vi "Lab Panel V5.25.1.vi"() -> ()   [LabVIEW 2013] (continued)
                    n1123 = Unbundle(w2133) -> ("CYCLE"=w2138:dbl)  [unwired: 2 out]
                    n1124 = Increment(x=w2130) -> (x+1=w2131:dbl)
                    n1125 = Greater Or Equal?(x=w2138, y=w2131) -> (x >= y?=w2140:bool)
                    n1126 = case shown="True" w2140 {
                      tunnel: w2135 -> [w2150 _]
                      tunnel: w2134 -> [w2149 _]
                      tunnel: w2133 -> [w2148 _]
                      tunnel: w2132 -> [w2147 _]
                      frame True {
                        n1127 = stacked-sequence {
                          tunnel: w2150 -> [w2154 _]
                          tunnel: w2149 -> [w2152 w2158]
                          tunnel: w2148 -> [_ w2161]
                          tunnel: w2147 -> [w2151 _]
                          frame #0 {
                            n1128 = Build Array(w2152) -> (w2155:string[])
                            n1129 = Build Array(w2154) -> (w2153:dbl[])
                            n1130 = TDMS Write(0:w2151, 5:"TEST PASS", 7:w2155, 9:w2153) -> (15:w2157:errorcluster)  [unwired: 2 in, 3 out]
                            n1131 = local write "data file error"(w2157) -> ()
                          }
                          frame #1 {
                            n1132 = Bundle(cluster=w2161, "STATUS"=w2158) -> (w2159:T4)  [unwired: 2 in]
                            n1133 = local write "RESULT LAB01-1"(TRUE) -> ()
                            n1134 = local write "DISP LAB01-1"(w2159) -> ()
                          }
                        }
                      }
                      frame False {
                      }
                    }
                  }
                }
              }
              frame #1 {
                # "LAB01-2"
                n1135 = Less?(x=w2162, y=2) -> (x < y?=w2165:bool)
                n1136 = local read "DISP LAB01-2"() -> (w2167:T4)
                n1137 = Unbundle(w2167) -> ("STATUS"=w2168:string)  [unwired: 2 out]
                n1138 = Equal?(x=w2168, y="RUN") -> (x = y?=w2164:bool)
                n1139 = And(x=w2164, y=w2165) -> (x .and. y?=w2163:bool)
                n1140 = case shown="True" w2163 {
                  tunnel: w2167 -> [_ w2173]
                  tunnel: w2162 -> [_ w2177]
                  frame False {
                  }
                  frame True {
                    n1141 = local read "SET LAB01-2"() -> (w2179:T5)
                    n1142 = local read "TDMS LAB01-2"() -> (w2172:refnum<k34>)
                    n1143 = Unbundle(w2179) -> ("CYCLES"=w2170:dbl, "T-RISE mins"=w2176:dbl)  [unwired: 3 out]
                    n1144 = case shown="\"T-RISE TEST\"" w2177 {
                      tunnel: w2176 -> [_ _ w2186]
                      tunnel: [w2181 w2183 w2186] -> w2175
                      tunnel: w2170 -> [w2181 w2183 _]
                      tunnel: ["CHART PASS" "CYCLE PASS" "T-RISE PASS"] -> w2174
                      frame "CHART TEST", Default {
                      }
                      frame "CYCLE TEST" {
                      }
                      frame "T-RISE TEST" {
                      }
                    }
                    n1145 = Unbundle(w2173) -> ("CYCLE"=w2178:dbl)  [unwired: 2 out]
                    n1146 = Increment(x=w2170) -> (x+1=w2171:dbl)
                    n1147 = Greater Or Equal?(x=w2178, y=w2171) -> (x >= y?=w2180:bool)
                    n1148 = case shown="True" w2180 {
                      tunnel: w2175 -> [w2190 _]
                      tunnel: w2174 -> [w2189 _]
                      tunnel: w2173 -> [w2188 _]
                      tunnel: w2172 -> [w2187 _]
                      frame True {
                        n1149 = stacked-sequence {
                          tunnel: w2190 -> [w2194 _]
                          tunnel: w2189 -> [w2192 w2198]
                          tunnel: w2188 -> [_ w2201]
                          tunnel: w2187 -> [w2191 _]
                          frame #0 {
                            n1150 = Build Array(w2192) -> (w2195:string[])
                            n1151 = Build Array(w2194) -> (w2193:dbl[])
                            n1152 = TDMS Write(0:w2191, 5:"TEST PASS", 7:w2195, 9:w2193) -> (15:w2197:errorcluster)  [unwired: 2 in, 3 out]
                            n1153 = local write "data file error"(w2197) -> ()
                          }
                          frame #1 {
                            n1154 = Bundle(cluster=w2201, "STATUS"=w2198) -> (w2199:T4)  [unwired: 2 in]
                            n1155 = local write "RESULT LAB01-2"(TRUE) -> ()
                            n1156 = local write "DISP LAB01-2"(w2199) -> ()
                          }
                        }
                      }
                      frame False {
                      }
                    }
                  }
                }
              }
              frame #2 {
                # "LAB02-1"
                n1157 = Less?(x=w2202, y=2) -> (x < y?=w2205:bool)
                n1158 = local read "DISP LAB02-1"() -> (w2207:T4)
                n1159 = Unbundle(w2207) -> ("STATUS"=w2208:string)  [unwired: 2 out]
                n1160 = Equal?(x=w2208, y="RUN") -> (x = y?=w2204:bool)
                n1161 = And(x=w2204, y=w2205) -> (x .and. y?=w2203:bool)
                n1162 = case shown="True" w2203 {
                  tunnel: w2207 -> [_ w2213]
                  tunnel: w2202 -> [_ w2217]
                  frame False {
                  }
                  frame True {
                    n1163 = local read "SET LAB02-1"() -> (w2219:T5)
                    n1164 = local read "TDMS LAB02-1"() -> (w2212:refnum<k34>)
                    n1165 = Unbundle(w2213) -> ("CYCLE"=w2218:dbl)  [unwired: 2 out]
                    n1166 = Unbundle(w2219) -> ("CYCLES"=w2210:dbl, "T-RISE mins"=w2216:dbl)  [unwired: 3 out]
                    n1167 = case shown="\"T-RISE TEST\"" w2217 {
                      tunnel: w2216 -> [_ _ w2226]
                      tunnel: [w2221 w2223 w2226] -> w2215
                      tunnel: w2210 -> [w2221 w2223 _]
                      tunnel: ["CHART PASS" "CYCLE PASS" "T-RISE PASS"] -> w2214
                      frame "CHART TEST", Default {
                      }
                      frame "CYCLE TEST" {
                      }
                      frame "T-RISE TEST" {
                      }
                    }
                    n1168 = Increment(x=w2210) -> (x+1=w2211:dbl)
                    n1169 = Greater Or Equal?(x=w2218, y=w2211) -> (x >= y?=w2220:bool)
                    n1170 = case shown="True" w2220 {
                      tunnel: w2215 -> [w2230 _]
                      tunnel: w2214 -> [w2229 _]
                      tunnel: w2213 -> [w2228 _]
                      tunnel: w2212 -> [w2227 _]
                      frame True {
                        n1171 = stacked-sequence {
                          tunnel: w2230 -> [w2234 _]
                          tunnel: w2229 -> [w2232 w2238]
                          tunnel: w2228 -> [_ w2241]
                          tunnel: w2227 -> [w2231 _]
                          frame #0 {
                            n1172 = Build Array(w2232) -> (w2235:string[])
                            n1173 = Build Array(w2234) -> (w2233:dbl[])
                            n1174 = TDMS Write(0:w2231, 5:"TEST PASS", 7:w2235, 9:w2233) -> (15:w2237:errorcluster)  [unwired: 2 in, 3 out]
                            n1175 = local write "data file error"(w2237) -> ()
                          }
                          frame #1 {
                            n1176 = Bundle(cluster=w2241, "STATUS"=w2238) -> (w2239:T4)  [unwired: 2 in]
                            n1177 = local write "RESULT LAB02-1"(TRUE) -> ()
                            n1178 = local write "DISP LAB02-1"(w2239) -> ()
                          }
                        }
                      }
                      frame False {
                      }
                    }
                  }
                }
              }
              frame #3 {
                # "LAB02-2"
                n1179 = Less?(x=w2242, y=2) -> (x < y?=w2245:bool)
                n1180 = local read "DISP LAB02-2"() -> (w2247:T4)
                n1181 = Unbundle(w2247) -> ("STATUS"=w2248:string)  [unwired: 2 out]
                n1182 = Equal?(x=w2248, y="RUN") -> (x = y?=w2244:bool)
                n1183 = And(x=w2244, y=w2245) -> (x .and. y?=w2243:bool)
                n1184 = case shown="True" w2243 {
                  tunnel: w2247 -> [_ w2253]
                  tunnel: w2242 -> [_ w2257]
                  frame False {
                  }
                  frame True {
                    n1185 = local read "SET LAB02-2"() -> (w2259:T5)
                    n1186 = local read "TDMS LAB02-2"() -> (w2252:refnum<k34>)
                    n1187 = Unbundle(w2253) -> ("CYCLE"=w2258:dbl)  [unwired: 2 out]
                    n1188 = Unbundle(w2259) -> ("CYCLES"=w2250:dbl, "T-RISE mins"=w2256:dbl)  [unwired: 3 out]
                    n1189 = case shown="\"T-RISE TEST\"" w2257 {
                      tunnel: w2256 -> [_ _ w2266]
                      tunnel: [w2261 w2263 w2266] -> w2255
                      tunnel: w2250 -> [w2261 w2263 _]
                      tunnel: ["CHART PASS" "CYCLE PASS" "T-RISE PASS"] -> w2254
                      frame "CHART TEST", Default {
                      }
                      frame "CYCLE TEST" {
                      }
                      frame "T-RISE TEST" {
                      }
                    }
                    n1190 = Increment(x=w2250) -> (x+1=w2251:dbl)
                    n1191 = Greater Or Equal?(x=w2258, y=w2251) -> (x >= y?=w2260:bool)
                    n1192 = case shown="True" w2260 {
                      tunnel: w2255 -> [w2270 _]
                      tunnel: w2254 -> [w2269 _]
                      tunnel: w2253 -> [w2268 _]
                      tunnel: w2252 -> [w2267 _]
                      frame True {
                        n1193 = stacked-sequence {
                          tunnel: w2270 -> [w2274 _]
                          tunnel: w2269 -> [w2272 w2278]
                          tunnel: w2268 -> [_ w2281]
                          tunnel: w2267 -> [w2271 _]
                          frame #0 {
                            n1194 = Build Array(w2272) -> (w2275:string[])
                            n1195 = Build Array(w2274) -> (w2273:dbl[])
                            n1196 = TDMS Write(0:w2271, 5:"TEST PASS", 7:w2275, 9:w2273) -> (15:w2277:errorcluster)  [unwired: 2 in, 3 out]
                            n1197 = local write "data file error"(w2277) -> ()
                          }
                          frame #1 {
                            n1198 = Bundle(cluster=w2281, "STATUS"=w2278) -> (w2279:T4)  [unwired: 2 in]
                            n1199 = local write "RESULT LAB02-2"(TRUE) -> ()
                            n1200 = local write "DISP LAB02-2"(w2279) -> ()
                          }
                        }
                      }
                      frame False {
                      }
                    }
                  }
                }
              }
              frame #4 {
                # "LAB03-1"
                n1201 = Less?(x=w2282, y=2) -> (x < y?=w2285:bool)
                n1202 = local read "DISP LAB03-1"() -> (w2287:T4)
                n1203 = Unbundle(w2287) -> ("STATUS"=w2288:string)  [unwired: 2 out]
                n1204 = Equal?(x=w2288, y="RUN") -> (x = y?=w2284:bool)
                n1205 = And(x=w2284, y=w2285) -> (x .and. y?=w2283:bool)
                n1206 = case shown="True" w2283 {
                  tunnel: w2287 -> [_ w2293]
                  tunnel: w2282 -> [_ w2297]
                  frame False {
                  }
                  frame True {
                    n1207 = local read "SET LAB03-1"() -> (w2299:T5)
                    n1208 = local read "TDMS LAB03-1"() -> (w2292:refnum<k34>)
                    n1209 = Unbundle(w2293) -> ("CYCLE"=w2298:dbl)  [unwired: 2 out]
                    n1210 = Unbundle(w2299) -> ("CYCLES"=w2290:dbl, "T-RISE mins"=w2296:dbl)  [unwired: 3 out]
                    n1211 = case shown="\"T-RISE TEST\"" w2297 {
                      tunnel: w2296 -> [_ _ w2306]
                      tunnel: [w2301 w2303 w2306] -> w2295
                      tunnel: w2290 -> [w2301 w2303 _]
                      tunnel: ["CHART PASS" "CYCLE PASS" "T-RISE PASS"] -> w2294
                      frame "CHART TEST", Default {
                      }
                      frame "CYCLE TEST" {
                      }
                      frame "T-RISE TEST" {
                      }
                    }
                    n1212 = Increment(x=w2290) -> (x+1=w2291:dbl)
                    n1213 = Greater Or Equal?(x=w2298, y=w2291) -> (x >= y?=w2300:bool)
                    n1214 = case shown="True" w2300 {
                      tunnel: w2295 -> [w2310 _]
                      tunnel: w2294 -> [w2309 _]
                      tunnel: w2293 -> [w2308 _]
                      tunnel: w2292 -> [w2307 _]
                      frame True {
                        n1215 = stacked-sequence {
                          tunnel: w2310 -> [w2314 _]
                          tunnel: w2309 -> [w2312 w2318]
                          tunnel: w2308 -> [_ w2321]
                          tunnel: w2307 -> [w2311 _]
                          frame #0 {
                            n1216 = Build Array(w2312) -> (w2315:string[])
                            n1217 = Build Array(w2314) -> (w2313:dbl[])
                            n1218 = TDMS Write(0:w2311, 5:"TEST PASS", 7:w2315, 9:w2313) -> (15:w2317:errorcluster)  [unwired: 2 in, 3 out]
                            n1219 = local write "data file error"(w2317) -> ()
                          }
                          frame #1 {
                            n1220 = Bundle(cluster=w2321, "STATUS"=w2318) -> (w2319:T4)  [unwired: 2 in]
                            n1221 = local write "RESULT LAB03-1"(TRUE) -> ()
                            n1222 = local write "DISP LAB03-1"(w2319) -> ()
                          }
                        }
                      }
                      frame False {
                      }
                    }
                  }
                }
              }
              frame #5 {
                # "LAB03-2"
                n1223 = Less?(x=w2322, y=2) -> (x < y?=w2325:bool)
                n1224 = local read "DISP LAB03-2"() -> (w2327:T4)
                n1225 = Unbundle(w2327) -> ("STATUS"=w2328:string)  [unwired: 2 out]
                n1226 = Equal?(x=w2328, y="RUN") -> (x = y?=w2324:bool)
                n1227 = And(x=w2324, y=w2325) -> (x .and. y?=w2323:bool)
                n1228 = case shown="True" w2323 {
                  tunnel: w2327 -> [_ w2333]
                  tunnel: w2322 -> [_ w2337]
                  frame False {
                  }
                  frame True {
                    n1229 = local read "SET LAB03-2"() -> (w2339:T5)
                    n1230 = local read "TDMS LAB03-2"() -> (w2332:refnum<k34>)
                    n1231 = Unbundle(w2333) -> ("CYCLE"=w2338:dbl)  [unwired: 2 out]
                    n1232 = Unbundle(w2339) -> ("CYCLES"=w2330:dbl, "T-RISE mins"=w2336:dbl)  [unwired: 3 out]
                    n1233 = case shown="\"T-RISE TEST\"" w2337 {
                      tunnel: w2336 -> [_ _ w2346]
                      tunnel: [w2341 w2343 w2346] -> w2335
                      tunnel: w2330 -> [w2341 w2343 _]
                      tunnel: ["CHART PASS" "CYCLE PASS" "T-RISE PASS"] -> w2334
                      frame "CHART TEST", Default {
                      }
                      frame "CYCLE TEST" {
                      }
                      frame "T-RISE TEST" {
                      }
                    }
                    n1234 = Increment(x=w2330) -> (x+1=w2331:dbl)
                    n1235 = Greater Or Equal?(x=w2338, y=w2331) -> (x >= y?=w2340:bool)
                    n1236 = case shown="True" w2340 {
                      tunnel: w2335 -> [w2350 _]
                      tunnel: w2334 -> [w2349 _]
                      tunnel: w2333 -> [w2348 _]
                      tunnel: w2332 -> [w2347 _]
                      frame True {
                        n1237 = stacked-sequence {
                          tunnel: w2350 -> [w2354 _]
                          tunnel: w2349 -> [w2352 w2358]
                          tunnel: w2348 -> [_ w2361]
                          tunnel: w2347 -> [w2351 _]
                          frame #0 {
                            n1238 = Build Array(w2352) -> (w2355:string[])
                            n1239 = Build Array(w2354) -> (w2353:dbl[])
                            n1240 = TDMS Write(0:w2351, 5:"TEST PASS", 7:w2355, 9:w2353) -> (15:w2357:errorcluster)  [unwired: 2 in, 3 out]
                            n1241 = local write "data file error"(w2357) -> ()
                          }
                          frame #1 {
                            n1242 = Bundle(cluster=w2361, "STATUS"=w2358) -> (w2359:T4)  [unwired: 2 in]
                            n1243 = local write "RESULT LAB03-2"(TRUE) -> ()
                            n1244 = local write "DISP LAB03-2"(w2359) -> ()
                          }
                        }
                      }
                      frame False {
                      }
                    }
                  }
                }
              }
              frame #6 {
                # "LAB04-1"
                n1245 = Less?(x=w2362, y=2) -> (x < y?=w2365:bool)
                n1246 = local read "DISP LAB04-1"() -> (w2367:T4)
                n1247 = Unbundle(w2367) -> ("STATUS"=w2368:string)  [unwired: 2 out]
                n1248 = Equal?(x=w2368, y="RUN") -> (x = y?=w2364:bool)
                n1249 = And(x=w2364, y=w2365) -> (x .and. y?=w2363:bool)
                n1250 = case shown="True" w2363 {
                  tunnel: w2367 -> [_ w2373]
                  tunnel: w2362 -> [_ w2377]
                  frame False {
                  }
                  frame True {
                    n1251 = local read "SET LAB04-1"() -> (w2379:T5)
                    n1252 = local read "TDMS LAB04-1"() -> (w2372:refnum<k34>)
                    n1253 = Unbundle(w2373) -> ("CYCLE"=w2378:dbl)  [unwired: 2 out]
                    n1254 = Unbundle(w2379) -> ("CYCLES"=w2370:dbl, "T-RISE mins"=w2376:dbl)  [unwired: 3 out]
                    n1255 = case shown="\"T-RISE TEST\"" w2377 {
                      tunnel: w2376 -> [_ _ w2386]
                      tunnel: [w2381 w2383 w2386] -> w2375
                      tunnel: w2370 -> [w2381 w2383 _]
                      tunnel: ["CHART PASS" "CYCLE PASS" "T-RISE PASS"] -> w2374
                      frame "CHART TEST", Default {
                      }
                      frame "CYCLE TEST" {
                      }
                      frame "T-RISE TEST" {
                      }
                    }
                    n1256 = Increment(x=w2370) -> (x+1=w2371:dbl)
                    n1257 = Greater Or Equal?(x=w2378, y=w2371) -> (x >= y?=w2380:bool)
                    n1258 = case shown="True" w2380 {
                      tunnel: w2375 -> [w2390 _]
                      tunnel: w2374 -> [w2389 _]
                      tunnel: w2373 -> [w2388 _]
                      tunnel: w2372 -> [w2387 _]
                      frame True {
                        n1259 = stacked-sequence {
                          tunnel: w2390 -> [w2394 _]
                          tunnel: w2389 -> [w2392 w2398]
                          tunnel: w2388 -> [_ w2401]
                          tunnel: w2387 -> [w2391 _]
                          frame #0 {
                            n1260 = Build Array(w2392) -> (w2395:string[])
                            n1261 = Build Array(w2394) -> (w2393:dbl[])
                            n1262 = TDMS Write(0:w2391, 5:"TEST PASS", 7:w2395, 9:w2393) -> (15:w2397:errorcluster)  [unwired: 2 in, 3 out]
                            n1263 = local write "data file error"(w2397) -> ()
                          }
                          frame #1 {
                            n1264 = Bundle(cluster=w2401, "STATUS"=w2398) -> (w2399:T4)  [unwired: 2 in]
                            n1265 = local write "RESULT LAB04-1"(TRUE) -> ()
                            n1266 = local write "DISP LAB04-1"(w2399) -> ()
                          }
                        }
                      }
                      frame False {
                      }
                    }
                  }
                }
              }
              frame #7 {
                # "LAB04-2"
                n1267 = Less?(x=w2402, y=2) -> (x < y?=w2405:bool)
                n1268 = local read "DISP LAB04-2"() -> (w2407:T4)
                n1269 = Unbundle(w2407) -> ("STATUS"=w2408:string)  [unwired: 2 out]
                n1270 = Equal?(x=w2408, y="RUN") -> (x = y?=w2404:bool)
                n1271 = And(x=w2404, y=w2405) -> (x .and. y?=w2403:bool)
                n1272 = case shown="True" w2403 {
                  tunnel: w2407 -> [_ w2413]
                  tunnel: w2402 -> [_ w2417]
                  frame False {
                  }
                  frame True {
                    n1273 = local read "SET LAB04-2"() -> (w2419:T5)
                    n1274 = local read "TDMS LAB04-2"() -> (w2412:refnum<k34>)
                    n1275 = Unbundle(w2413) -> ("CYCLE"=w2418:dbl)  [unwired: 2 out]
                    n1276 = Unbundle(w2419) -> ("CYCLES"=w2410:dbl, "T-RISE mins"=w2416:dbl)  [unwired: 3 out]
                    n1277 = case shown="\"T-RISE TEST\"" w2417 {
                      tunnel: w2416 -> [_ _ w2426]
                      tunnel: [w2421 w2423 w2426] -> w2415
                      tunnel: w2410 -> [w2421 w2423 _]
                      tunnel: ["CHART PASS" "CYCLE PASS" "T-RISE PASS"] -> w2414
                      frame "CHART TEST", Default {
                      }
                      frame "CYCLE TEST" {
                      }
                      frame "T-RISE TEST" {
                      }
                    }
                    n1278 = Increment(x=w2410) -> (x+1=w2411:dbl)
                    n1279 = Greater Or Equal?(x=w2418, y=w2411) -> (x >= y?=w2420:bool)
                    n1280 = case shown="True" w2420 {
                      tunnel: w2415 -> [w2430 _]
                      tunnel: w2414 -> [w2429 _]
                      tunnel: w2413 -> [w2428 _]
                      tunnel: w2412 -> [w2427 _]
                      frame True {
                        n1281 = stacked-sequence {
                          tunnel: w2430 -> [w2434 _]
                          tunnel: w2429 -> [w2432 w2438]
                          tunnel: w2428 -> [_ w2441]
                          tunnel: w2427 -> [w2431 _]
                          frame #0 {
                            n1282 = Build Array(w2432) -> (w2435:string[])
                            n1283 = Build Array(w2434) -> (w2433:dbl[])
                            n1284 = TDMS Write(0:w2431, 5:"TEST PASS", 7:w2435, 9:w2433) -> (15:w2437:errorcluster)  [unwired: 2 in, 3 out]
                            n1285 = local write "data file error"(w2437) -> ()
                          }
                          frame #1 {
                            n1286 = Bundle(cluster=w2441, "STATUS"=w2438) -> (w2439:T4)  [unwired: 2 in]
                            n1287 = local write "RESULT LAB04-2"(TRUE) -> ()
                            n1288 = local write "DISP LAB04-2"(w2439) -> ()
                          }
                        }
                      }
                      frame False {
                      }
                    }
                  }
                }
              }
              frame #8 {
                # "LAB05-1"
                n1289 = Less?(x=w2442, y=2) -> (x < y?=w2445:bool)
                n1290 = local read "DISP LAB05-1"() -> (w2447:T4)
                n1291 = Unbundle(w2447) -> ("STATUS"=w2448:string)  [unwired: 2 out]
                n1292 = Equal?(x=w2448, y="RUN") -> (x = y?=w2444:bool)
                n1293 = And(x=w2444, y=w2445) -> (x .and. y?=w2443:bool)
                n1294 = case shown="True" w2443 {
                  tunnel: w2447 -> [_ w2453]
                  tunnel: w2442 -> [_ w2457]
                  frame False {
                  }
                  frame True {
                    n1295 = local read "SET LAB05-1"() -> (w2459:T5)
                    n1296 = local read "TDMS LAB05-1"() -> (w2452:refnum<k34>)
                    n1297 = Unbundle(w2453) -> ("CYCLE"=w2458:dbl)  [unwired: 2 out]
                    n1298 = Unbundle(w2459) -> ("CYCLES"=w2450:dbl, "T-RISE mins"=w2456:dbl)  [unwired: 3 out]
                    n1299 = case shown="\"T-RISE TEST\"" w2457 {
                      tunnel: w2456 -> [_ _ w2466]
                      tunnel: [w2461 w2463 w2466] -> w2455
                      tunnel: w2450 -> [w2461 w2463 _]
                      tunnel: ["CHART PASS" "CYCLE PASS" "T-RISE PASS"] -> w2454
                      frame "CHART TEST", Default {
                      }
                      frame "CYCLE TEST" {
                      }
                      frame "T-RISE TEST" {
                      }
                    }
                    n1300 = Increment(x=w2450) -> (x+1=w2451:dbl)
                    n1301 = Greater Or Equal?(x=w2458, y=w2451) -> (x >= y?=w2460:bool)
                    n1302 = case shown="True" w2460 {
                      tunnel: w2455 -> [w2470 _]
                      tunnel: w2454 -> [w2469 _]
                      tunnel: w2453 -> [w2468 _]
                      tunnel: w2452 -> [w2467 _]
                      frame True {
                        n1303 = stacked-sequence {
                          tunnel: w2470 -> [w2474 _]
                          tunnel: w2469 -> [w2472 w2478]
                          tunnel: w2468 -> [_ w2481]
                          tunnel: w2467 -> [w2471 _]
                          frame #0 {
                            n1304 = Build Array(w2472) -> (w2475:string[])
                            n1305 = Build Array(w2474) -> (w2473:dbl[])
                            n1306 = TDMS Write(0:w2471, 5:"TEST PASS", 7:w2475, 9:w2473) -> (15:w2477:errorcluster)  [unwired: 2 in, 3 out]
                            n1307 = local write "data file error"(w2477) -> ()
                          }
                          frame #1 {
                            n1308 = Bundle(cluster=w2481, "STATUS"=w2478) -> (w2479:T4)  [unwired: 2 in]
                            n1309 = local write "RESULT LAB05-1"(TRUE) -> ()
                            n1310 = local write "DISP LAB05-1"(w2479) -> ()
                          }
                        }
                      }
                      frame False {
                      }
                    }
                  }
                }
              }
              frame #9 {
                # "LAB05-2"
                n1311 = Less?(x=w2482, y=2) -> (x < y?=w2485:bool)
                n1312 = local read "DISP LAB05-2"() -> (w2487:T4)
                n1313 = Unbundle(w2487) -> ("STATUS"=w2488:string)  [unwired: 2 out]
                n1314 = Equal?(x=w2488, y="RUN") -> (x = y?=w2484:bool)
                n1315 = And(x=w2484, y=w2485) -> (x .and. y?=w2483:bool)
                n1316 = case shown="True" w2483 {
                  tunnel: w2487 -> [_ w2493]
                  tunnel: w2482 -> [_ w2497]
                  frame False {
                  }
                  frame True {
                    n1317 = local read "SET LAB05-2"() -> (w2499:T5)
                    n1318 = local read "TDMS LAB05-2"() -> (w2492:refnum<k34>)
                    n1319 = Unbundle(w2493) -> ("CYCLE"=w2498:dbl)  [unwired: 2 out]
                    n1320 = Unbundle(w2499) -> ("CYCLES"=w2490:dbl, "T-RISE mins"=w2496:dbl)  [unwired: 3 out]
                    n1321 = case shown="\"T-RISE TEST\"" w2497 {
                      tunnel: w2496 -> [_ _ w2506]
                      tunnel: [w2501 w2503 w2506] -> w2495
                      tunnel: w2490 -> [w2501 w2503 _]
                      tunnel: ["CHART PASS" "CYCLE PASS" "T-RISE PASS"] -> w2494
                      frame "CHART TEST", Default {
                      }
                      frame "CYCLE TEST" {
                      }
                      frame "T-RISE TEST" {
                      }
                    }
                    n1322 = Increment(x=w2490) -> (x+1=w2491:dbl)
                    n1323 = Greater Or Equal?(x=w2498, y=w2491) -> (x >= y?=w2500:bool)
                    n1324 = case shown="True" w2500 {
                      tunnel: w2495 -> [w2510 _]
                      tunnel: w2494 -> [w2509 _]
                      tunnel: w2493 -> [w2508 _]
                      tunnel: w2492 -> [w2507 _]
                      frame True {
                        n1325 = stacked-sequence {
                          tunnel: w2510 -> [w2514 _]
                          tunnel: w2509 -> [w2512 w2518]
                          tunnel: w2508 -> [_ w2521]
                          tunnel: w2507 -> [w2511 _]
                          frame #0 {
                            n1326 = Build Array(w2512) -> (w2515:string[])
                            n1327 = Build Array(w2514) -> (w2513:dbl[])
                            n1328 = TDMS Write(0:w2511, 5:"TEST PASS", 7:w2515, 9:w2513) -> (15:w2517:errorcluster)  [unwired: 2 in, 3 out]
                            n1329 = local write "data file error"(w2517) -> ()
                          }
                          frame #1 {
                            n1330 = Bundle(cluster=w2521, "STATUS"=w2518) -> (w2519:T4)  [unwired: 2 in]
                            n1331 = local write "RESULT LAB05-2"(TRUE) -> ()
                            n1332 = local write "DISP LAB05-2"(w2519) -> ()
                          }
                        }
                      }
                      frame False {
                      }
                    }
                  }
                }
              }
            }
          }
          frame #6 {
            # "check if test cycles reached for temperature rise test"
            n1333 = stacked-sequence {
              tunnel: w2551 -> [_ _ _ _ _ _ _ _ _ _]
              tunnel: w2550 -> [_ _ _ _ _ _ _ _ _ _]
              tunnel: w2549 -> [_ _ _ _ _ _ _ _ _ _]
              tunnel: w2548 -> [_ _ _ _ _ _ _ _ _ _]
              tunnel: w2547 -> [_ _ _ _ _ _ _ _ _ _]
              tunnel: w2546 -> [_ _ _ _ _ _ _ _ _ _]
              tunnel: w2545 -> [_ _ _ _ _ _ _ _ _ _]
              tunnel: w2544 -> [_ _ _ _ _ _ _ _ _ _]
              tunnel: w2543 -> [_ _ _ _ _ _ _ _ _ _]
              tunnel: w2542 -> [_ _ _ _ _ _ _ _ _ _]
              tunnel: w2541 -> [w2557 _ _ _ _ _ _ _ _ _]
              tunnel: w2531 -> [w2552 _ _ _ _ _ _ _ _ _]
              tunnel: w2540 -> [_ w2583 _ _ _ _ _ _ _ _]
              tunnel: w2539 -> [_ _ w2613 _ _ _ _ _ _ _]
              tunnel: w2538 -> [_ _ _ w2643 _ _ _ _ _ _]
              tunnel: w2537 -> [_ _ _ _ w2673 _ _ _ _ _]
              tunnel: w2536 -> [_ _ _ _ _ w2703 _ _ _ _]
              tunnel: w2535 -> [_ _ _ _ _ _ w2733 _ _ _]
              tunnel: w2534 -> [_ _ _ _ _ _ _ w2763 _ _]
              tunnel: w2533 -> [_ _ _ _ _ _ _ _ w2793 _]
              tunnel: w2532 -> [_ _ _ _ _ _ _ _ _ w2823]
              tunnel: w2530 -> [_ w2582 _ _ _ _ _ _ _ _]
              tunnel: w2529 -> [_ _ w2612 _ _ _ _ _ _ _]
              tunnel: w2528 -> [_ _ _ w2642 _ _ _ _ _ _]
              tunnel: w2527 -> [_ _ _ _ w2672 _ _ _ _ _]
              tunnel: w2526 -> [_ _ _ _ _ w2702 _ _ _ _]
              tunnel: w2525 -> [_ _ _ _ _ _ w2732 _ _ _]
              tunnel: w2524 -> [_ _ _ _ _ _ _ w2762 _ _]
              tunnel: w2523 -> [_ _ _ _ _ _ _ _ w2792 _]
              tunnel: w2522 -> [_ _ _ _ _ _ _ _ _ w2822]
              frame #0 {
                # "LAB01-1"
                n1334 = Equal?(x=w2557, y=2) -> (x = y?=w2555:bool)
                n1335 = local read "DISP LAB01-1"() -> (w2558:T4)
                n1336 = Unbundle(w2558) -> ("STATUS"=w2559:string)  [unwired: 2 out]
                n1337 = Equal?(x=w2559, y="RUN") -> (x = y?=w2554:bool)
                n1338 = And(x=w2554, y=w2555) -> (x .and. y?=w2553:bool)
                n1339 = case shown="True" w2553 {
                  tunnel: w2558 -> [_ w2562]
                  tunnel: w2552 -> [_ w2565]
                  frame False {
                  }
                  frame True {
                    n1340 = local read "SET LAB01-1"() -> (w2564:T5)
                    n1341 = local read "TDMS LAB01-1"() -> (w2561:refnum<k34>)
                    n1342 = Unbundle(w2562) -> ("CYCLE"=w2566:dbl)  [unwired: 2 out]
                    n1343 = Unbundle(w2564) -> ("T-RISE mins"=w2563:dbl)  [unwired: 4 out]
                    n1344 = Greater Or Equal?(x=w2566, y=w2565) -> (x >= y?=w2567:bool)
                    n1345 = case shown="True" w2567 {
                      tunnel: w2563 -> [w2570 _]
                      tunnel: w2562 -> [w2569 _]
                      tunnel: w2561 -> [w2568 _]
                      frame True {
                        n1346 = stacked-sequence {
                          tunnel: w2570 -> [w2573 _]
                          tunnel: w2569 -> [_ w2578]
                          tunnel: w2568 -> [w2571 _]
                          frame #0 {
                            n1347 = Build Array("T-RISE") -> (w2575:string[])
                            n1348 = Build Array(w2573) -> (w2574:dbl[])
                            n1349 = TDMS Write(0:w2571, 5:"TEST PASS", 7:w2575, 9:w2574) -> (15:w2577:errorcluster)  [unwired: 2 in, 3 out]
                            n1350 = local write "data file error"(w2577) -> ()
                          }
                          frame #1 {
                            n1351 = Bundle(cluster=w2578, "STATUS"="T-RISE PASS") -> (w2580:T4)  [unwired: 2 in]
                            n1352 = local write "RESULT LAB01-1"(TRUE) -> ()
                            n1353 = local write "DISP LAB01-1"(w2580) -> ()
                          }
                        }
                      }
                      frame False {
                      }
                    }
                  }
                }
              }
              frame #1 {
                # "LAB01-2"
                n1354 = Equal?(x=w2583, y=2) -> (x = y?=w2586:bool)
                n1355 = local read "DISP LAB01-2"() -> (w2588:T4)
                n1356 = Unbundle(w2588) -> ("STATUS"=w2589:string)  [unwired: 2 out]
                n1357 = Equal?(x=w2589, y="RUN") -> (x = y?=w2585:bool)
                n1358 = And(x=w2585, y=w2586) -> (x .and. y?=w2584:bool)
                n1359 = case shown="True" w2584 {
                  tunnel: w2588 -> [_ w2592]
                  tunnel: w2582 -> [_ w2595]
                  frame False {
                  }
                  frame True {
                    n1360 = local read "SET LAB01-2"() -> (w2594:T5)
                    n1361 = local read "TDMS LAB01-2"() -> (w2591:refnum<k34>)
                    n1362 = Unbundle(w2592) -> ("CYCLE"=w2596:dbl)  [unwired: 2 out]
                    n1363 = Unbundle(w2594) -> ("T-RISE mins"=w2593:dbl)  [unwired: 4 out]
                    n1364 = Greater Or Equal?(x=w2596, y=w2595) -> (x >= y?=w2597:bool)
                    n1365 = case shown="True" w2597 {
                      tunnel: w2593 -> [w2600 _]
                      tunnel: w2592 -> [w2599 _]
                      tunnel: w2591 -> [w2598 _]
                      frame True {
                        n1366 = stacked-sequence {
                          tunnel: w2600 -> [w2603 _]
                          tunnel: w2599 -> [_ w2608]
                          tunnel: w2598 -> [w2601 _]
                          frame #0 {
                            n1367 = Build Array("T-RISE") -> (w2605:string[])
                            n1368 = Build Array(w2603) -> (w2604:dbl[])
                            n1369 = TDMS Write(0:w2601, 5:"TEST PASS", 7:w2605, 9:w2604) -> (15:w2607:errorcluster)  [unwired: 2 in, 3 out]
                            n1370 = local write "data file error"(w2607) -> ()
                          }
                          frame #1 {
                            n1371 = Bundle(cluster=w2608, "STATUS"="T-RISE PASS") -> (w2610:T4)  [unwired: 2 in]
                            n1372 = local write "RESULT LAB01-2"(TRUE) -> ()
                            n1373 = local write "DISP LAB01-2"(w2610) -> ()
                          }
                        }
                      }
                      frame False {
                      }
                    }
                  }
                }
              }
              frame #2 {
                # "LAB02-1"
                n1374 = Equal?(x=w2613, y=2) -> (x = y?=w2616:bool)
                n1375 = local read "DISP LAB02-1"() -> (w2618:T4)
                n1376 = Unbundle(w2618) -> ("STATUS"=w2619:string)  [unwired: 2 out]
                n1377 = Equal?(x=w2619, y="RUN") -> (x = y?=w2615:bool)
                n1378 = And(x=w2615, y=w2616) -> (x .and. y?=w2614:bool)
                n1379 = case shown="True" w2614 {
                  tunnel: w2618 -> [_ w2622]
                  tunnel: w2612 -> [_ w2625]
                  frame False {
                  }
                  frame True {
                    n1380 = local read "SET LAB02-1"() -> (w2624:T5)
                    n1381 = local read "TDMS LAB02-1"() -> (w2621:refnum<k34>)
                    n1382 = Unbundle(w2622) -> ("CYCLE"=w2626:dbl)  [unwired: 2 out]
                    n1383 = Unbundle(w2624) -> ("T-RISE mins"=w2623:dbl)  [unwired: 4 out]
                    n1384 = Greater Or Equal?(x=w2626, y=w2625) -> (x >= y?=w2627:bool)
                    n1385 = case shown="True" w2627 {
                      tunnel: w2623 -> [w2630 _]
                      tunnel: w2622 -> [w2629 _]
                      tunnel: w2621 -> [w2628 _]
                      frame True {
                        n1386 = stacked-sequence {
                          tunnel: w2630 -> [w2633 _]
                          tunnel: w2629 -> [_ w2638]
                          tunnel: w2628 -> [w2631 _]
                          frame #0 {
                            n1387 = Build Array("T-RISE") -> (w2635:string[])
                            n1388 = Build Array(w2633) -> (w2634:dbl[])
                            n1389 = TDMS Write(0:w2631, 5:"TEST PASS", 7:w2635, 9:w2634) -> (15:w2637:errorcluster)  [unwired: 2 in, 3 out]
                            n1390 = local write "data file error"(w2637) -> ()
                          }
                          frame #1 {
                            n1391 = Bundle(cluster=w2638, "STATUS"="T-RISE PASS") -> (w2640:T4)  [unwired: 2 in]
                            n1392 = local write "RESULT LAB02-1"(TRUE) -> ()
                            n1393 = local write "DISP LAB02-1"(w2640) -> ()
                          }
                        }
                      }
                      frame False {
                      }
                    }
                  }
                }
              }
              frame #3 {
                # "LAB02-2"
                n1394 = Equal?(x=w2643, y=2) -> (x = y?=w2646:bool)
                n1395 = local read "DISP LAB02-2"() -> (w2648:T4)
                n1396 = Unbundle(w2648) -> ("STATUS"=w2649:string)  [unwired: 2 out]
                n1397 = Equal?(x=w2649, y="RUN") -> (x = y?=w2645:bool)
                n1398 = And(x=w2645, y=w2646) -> (x .and. y?=w2644:bool)
                n1399 = case shown="True" w2644 {
                  tunnel: w2648 -> [_ w2652]
                  tunnel: w2642 -> [_ w2655]
                  frame False {
                  }
                  frame True {
                    n1400 = local read "SET LAB02-2"() -> (w2654:T5)
                    n1401 = local read "TDMS LAB02-2"() -> (w2651:refnum<k34>)
                    n1402 = Unbundle(w2652) -> ("CYCLE"=w2656:dbl)  [unwired: 2 out]
                    n1403 = Unbundle(w2654) -> ("T-RISE mins"=w2653:dbl)  [unwired: 4 out]
                    n1404 = Greater Or Equal?(x=w2656, y=w2655) -> (x >= y?=w2657:bool)
                    n1405 = case shown="True" w2657 {
                      tunnel: w2653 -> [w2660 _]
                      tunnel: w2652 -> [w2659 _]
                      tunnel: w2651 -> [w2658 _]
                      frame True {
                        n1406 = stacked-sequence {
                          tunnel: w2660 -> [w2663 _]
                          tunnel: w2659 -> [_ w2668]
                          tunnel: w2658 -> [w2661 _]
                          frame #0 {
                            n1407 = Build Array("T-RISE") -> (w2665:string[])
                            n1408 = Build Array(w2663) -> (w2664:dbl[])
                            n1409 = TDMS Write(0:w2661, 5:"TEST PASS", 7:w2665, 9:w2664) -> (15:w2667:errorcluster)  [unwired: 2 in, 3 out]
                            n1410 = local write "data file error"(w2667) -> ()
                          }
                          frame #1 {
                            n1411 = Bundle(cluster=w2668, "STATUS"="T-RISE PASS") -> (w2670:T4)  [unwired: 2 in]
                            n1412 = local write "RESULT LAB02-2"(TRUE) -> ()
                            n1413 = local write "DISP LAB02-2"(w2670) -> ()
                          }
                        }
                      }
                      frame False {
                      }
                    }
                  }
                }
              }
              frame #4 {
                # "LAB03-1"
                n1414 = Equal?(x=w2673, y=2) -> (x = y?=w2676:bool)
                n1415 = local read "DISP LAB03-1"() -> (w2678:T4)
                n1416 = Unbundle(w2678) -> ("STATUS"=w2679:string)  [unwired: 2 out]
                n1417 = Equal?(x=w2679, y="RUN") -> (x = y?=w2675:bool)
                n1418 = And(x=w2675, y=w2676) -> (x .and. y?=w2674:bool)
                n1419 = case shown="True" w2674 {
                  tunnel: w2678 -> [_ w2682]
                  tunnel: w2672 -> [_ w2685]
                  frame False {
                  }
                  frame True {
                    n1420 = local read "SET LAB03-1"() -> (w2684:T5)
                    n1421 = local read "TDMS LAB03-1"() -> (w2681:refnum<k34>)
                    n1422 = Unbundle(w2682) -> ("CYCLE"=w2686:dbl)  [unwired: 2 out]
                    n1423 = Unbundle(w2684) -> ("T-RISE mins"=w2683:dbl)  [unwired: 4 out]
                    n1424 = Greater Or Equal?(x=w2686, y=w2685) -> (x >= y?=w2687:bool)
                    n1425 = case shown="True" w2687 {
                      tunnel: w2683 -> [w2690 _]
                      tunnel: w2682 -> [w2689 _]
                      tunnel: w2681 -> [w2688 _]
                      frame True {
                        n1426 = stacked-sequence {
                          tunnel: w2690 -> [w2693 _]
                          tunnel: w2689 -> [_ w2698]
                          tunnel: w2688 -> [w2691 _]
                          frame #0 {
                            n1427 = Build Array("T-RISE") -> (w2695:string[])
                            n1428 = Build Array(w2693) -> (w2694:dbl[])
                            n1429 = TDMS Write(0:w2691, 5:"TEST PASS", 7:w2695, 9:w2694) -> (15:w2697:errorcluster)  [unwired: 2 in, 3 out]
                            n1430 = local write "data file error"(w2697) -> ()
                          }
                          frame #1 {
                            n1431 = Bundle(cluster=w2698, "STATUS"="T-RISE PASS") -> (w2700:T4)  [unwired: 2 in]
                            n1432 = local write "RESULT LAB03-1"(TRUE) -> ()
                            n1433 = local write "DISP LAB03-1"(w2700) -> ()
                          }
                        }
                      }
                      frame False {
                      }
                    }
                  }
                }
              }
              frame #5 {
                # "LAB03-2"
                n1434 = Equal?(x=w2703, y=2) -> (x = y?=w2706:bool)
                n1435 = local read "DISP LAB03-2"() -> (w2708:T4)
                n1436 = Unbundle(w2708) -> ("STATUS"=w2709:string)  [unwired: 2 out]
                n1437 = Equal?(x=w2709, y="RUN") -> (x = y?=w2705:bool)
                n1438 = And(x=w2705, y=w2706) -> (x .and. y?=w2704:bool)
                n1439 = case shown="True" w2704 {
                  tunnel: w2708 -> [_ w2712]
                  tunnel: w2702 -> [_ w2715]
                  frame False {
                  }
                  frame True {
                    n1440 = local read "SET LAB03-2"() -> (w2714:T5)
                    n1441 = local read "TDMS LAB03-2"() -> (w2711:refnum<k34>)
                    n1442 = Unbundle(w2712) -> ("CYCLE"=w2716:dbl)  [unwired: 2 out]
                    n1443 = Unbundle(w2714) -> ("T-RISE mins"=w2713:dbl)  [unwired: 4 out]
                    n1444 = Greater Or Equal?(x=w2716, y=w2715) -> (x >= y?=w2717:bool)
                    n1445 = case shown="True" w2717 {
                      tunnel: w2713 -> [w2720 _]
                      tunnel: w2712 -> [w2719 _]
                      tunnel: w2711 -> [w2718 _]
                      frame True {
                        n1446 = stacked-sequence {
                          tunnel: w2720 -> [w2723 _]
                          tunnel: w2719 -> [_ w2728]
                          tunnel: w2718 -> [w2721 _]
                          frame #0 {
                            n1447 = Build Array("T-RISE") -> (w2725:string[])
                            n1448 = Build Array(w2723) -> (w2724:dbl[])
                            n1449 = TDMS Write(0:w2721, 5:"TEST PASS", 7:w2725, 9:w2724) -> (15:w2727:errorcluster)  [unwired: 2 in, 3 out]
                            n1450 = local write "data file error"(w2727) -> ()
                          }
                          frame #1 {
                            n1451 = Bundle(cluster=w2728, "STATUS"="T-RISE PASS") -> (w2730:T4)  [unwired: 2 in]
                            n1452 = local write "RESULT LAB03-2"(TRUE) -> ()
                            n1453 = local write "DISP LAB03-2"(w2730) -> ()
                          }
                        }
                      }
                      frame False {
                      }
                    }
                  }
                }
              }
              frame #6 {
                # "LAB04-1"
                n1454 = Equal?(x=w2733, y=2) -> (x = y?=w2736:bool)
                n1455 = local read "DISP LAB04-1"() -> (w2738:T4)
                n1456 = Unbundle(w2738) -> ("STATUS"=w2739:string)  [unwired: 2 out]
                n1457 = Equal?(x=w2739, y="RUN") -> (x = y?=w2735:bool)
                n1458 = And(x=w2735, y=w2736) -> (x .and. y?=w2734:bool)
                n1459 = case shown="True" w2734 {
                  tunnel: w2738 -> [_ w2742]
                  tunnel: w2732 -> [_ w2745]
                  frame False {
                  }
                  frame True {
                    n1460 = local read "SET LAB04-1"() -> (w2744:T5)
                    n1461 = local read "TDMS LAB04-1"() -> (w2741:refnum<k34>)
                    n1462 = Unbundle(w2742) -> ("CYCLE"=w2746:dbl)  [unwired: 2 out]
                    n1463 = Unbundle(w2744) -> ("T-RISE mins"=w2743:dbl)  [unwired: 4 out]
                    n1464 = Greater Or Equal?(x=w2746, y=w2745) -> (x >= y?=w2747:bool)
                    n1465 = case shown="True" w2747 {
                      tunnel: w2743 -> [w2750 _]
                      tunnel: w2742 -> [w2749 _]
                      tunnel: w2741 -> [w2748 _]
                      frame True {
                        n1466 = stacked-sequence {
                          tunnel: w2750 -> [w2753 _]
                          tunnel: w2749 -> [_ w2758]
                          tunnel: w2748 -> [w2751 _]
                          frame #0 {
                            n1467 = Build Array("T-RISE") -> (w2755:string[])
                            n1468 = Build Array(w2753) -> (w2754:dbl[])
                            n1469 = TDMS Write(0:w2751, 5:"TEST PASS", 7:w2755, 9:w2754) -> (15:w2757:errorcluster)  [unwired: 2 in, 3 out]
                            n1470 = local write "data file error"(w2757) -> ()
                          }
                          frame #1 {
                            n1471 = Bundle(cluster=w2758, "STATUS"="T-RISE PASS") -> (w2760:T4)  [unwired: 2 in]
                            n1472 = local write "RESULT LAB04-1"(TRUE) -> ()
                            n1473 = local write "DISP LAB04-1"(w2760) -> ()
                          }
                        }
                      }
                      frame False {
                      }
                    }
                  }
                }
              }
              frame #7 {
                # "LAB04-2"
                n1474 = Equal?(x=w2763, y=2) -> (x = y?=w2766:bool)
                n1475 = local read "DISP LAB04-2"() -> (w2768:T4)
                n1476 = Unbundle(w2768) -> ("STATUS"=w2769:string)  [unwired: 2 out]
                n1477 = Equal?(x=w2769, y="RUN") -> (x = y?=w2765:bool)
                n1478 = And(x=w2765, y=w2766) -> (x .and. y?=w2764:bool)
                n1479 = case shown="True" w2764 {
                  tunnel: w2768 -> [_ w2772]
                  tunnel: w2762 -> [_ w2775]
                  frame False {
                  }
                  frame True {
                    n1480 = local read "SET LAB04-2"() -> (w2774:T5)
